vi "cDAQ_VI_Leo_Modified.vi"() -> ()   [LabVIEW 2022 SP3]
uses:
  <vilib>/Analysis/3filter.llb/Filter Passband Type.ctl
  <vilib>/Analysis/baseanly.llb/Mean (DBL).vi
  <vilib>/DAQmx/read.llb/DAQmx Read (Analog 1D Wfm NChan NSamp).vi
  STOP_GLOBAL.vi
  <vilib>/addons/control/pid/pid.llb/PID Lead-Lag (DBL).vi
  <vilib>/addons/control/pid/pid.llb/PID (DBL).vi
  <vilib>/DAQmx/configure/timing.llb/DAQmx Timing (Sample Clock).vi
  <vilib>/DAQmx/miscellaneous.llb/DAQmx Fill In Error Info.vi
  <vilib>/Analysis/3filter.llb/Butterworth Filter (DBL).vi
  <vilib>/Analysis/NI_AALBase.lvlib
  <vilib>/addons/control/pid/NI_PID_pid.lvlib
panel:
  out "Supply Pressure Mean":dbl format="%0.2f"
  out "Servo Voltage Input 3":cluster{dbl[], "Filtered X":dbl[]}[](graph)
  out "Servo Voltage Input 2":cluster{dbl[], dbl[]}(graph)
  out "Test":dynamicdata(graph)
  out "output":dbl format="%.2f"
  out "Voltage Input":dynamicdata(graph)
  out "Servo Voltage Input":cluster{dbl[], dbl[]}(graph)
  out "Elapsed Time (s)":dbl
  in  "Tab Control":T1(tab)
  in  "Channel Array":dbl[](array[numeric]) format="%_3g"
  out "error out 5":errorcluster
  in  "stop":bool
  out "Output":dbl(slide) scale=0.0..5.067
  out "elapsed time (s)":dbl format="%.3f"
  in  "reinitialize? (F)":bool
  out "Waveform Chart 2":cluster{"setpoint":dbl, dbl}(graph) caption="Waveform Chart"
  out "XY Graph":cluster{dbl[], dbl[]}[](graph)
  out "error out":errorcluster
  out "Steps on Needle 3":dbl[](array[numeric])
  in  "Error":dbl
  in  "Scaling Factor":dbl
  in  "x0":dbl
  in  "PID gains":T2={"proportional gain (Kc)"=1.0, "integral time (Ti, min)"=0.01, "derivative time (Td, min)"=0.0} {"derivative time (Td, min)" format="%.3f"; "integral time (Ti, min)" format="%.3f"; "proportional gain (Kc)" format="%.3f"}
  out "element":dbl
  out "Process variable":dbl
  out "Setpoint":dbl
  in  "setpoint profile":cluster{"time (s)":dbl, "setpoint":dbl}[](array[cluster]) {"setpoint" format="%.2f"; "time (s)" format="%.3f"}
  out "Steps on Servo":dbl[](array[numeric])
  out "Elapsed Time (s) 2":dbl caption="Elapsed Time (s)"
  out "HAS 3 SECONDS PASSED?":bool
  in  "PRESS TO START":bool
  out "All Channel Graph":cluster{dbl[], dbl[]}[](graph)
  out "Thrust":cluster{dbl[], dbl[]}(graph)
  out "Chamber Pressure":cluster{dbl[], dbl[]}(graph)
  out "Supply Pressure":cluster{dbl[], dbl[]}(graph)
  out "MassFlow":cluster{dbl[], dbl[]}(graph)
  out "Temperature":cluster{dbl[], dbl[]}(graph)
  out "error out 3":errorcluster caption="error out"
  out "error out 2":errorcluster
  in  "rate":dbl=1000.0 format="%0.2f"
  in  "number of samples":i32=100
  in  "File Format":string
  in  "File Name Out":string
  in  "Data Collection Folder":path
  out "Temperature":dynamicdata(graph)
  out "Numeric 2":i32
  out "Thrust lb":dynamicdata(graph)
  in  "Types of Testing":enum32{"Test Firing", "Cold Flow Rig"}(tab)
  out "Saving Data":bool
  out "Filename Out":path
  in  "Collect Data?":bool=TRUE caption="Enable"
  in  "Collect Data? 2":bool=TRUE caption="Enable"
  out "Saving Data":bool
  out "Filename Out":path
  out "Supply Pressure PSI":dynamicdata(graph)
  out "Mass Flow L/min":dynamicdata(graph)
  out "Chamber Pressure":dynamicdata(graph)
  # "Control Loop"
  # "DATA LOGGING INFORMATION"
  # "ANALOG VOLTAGE OUTPUT"
  # "RESULTS"
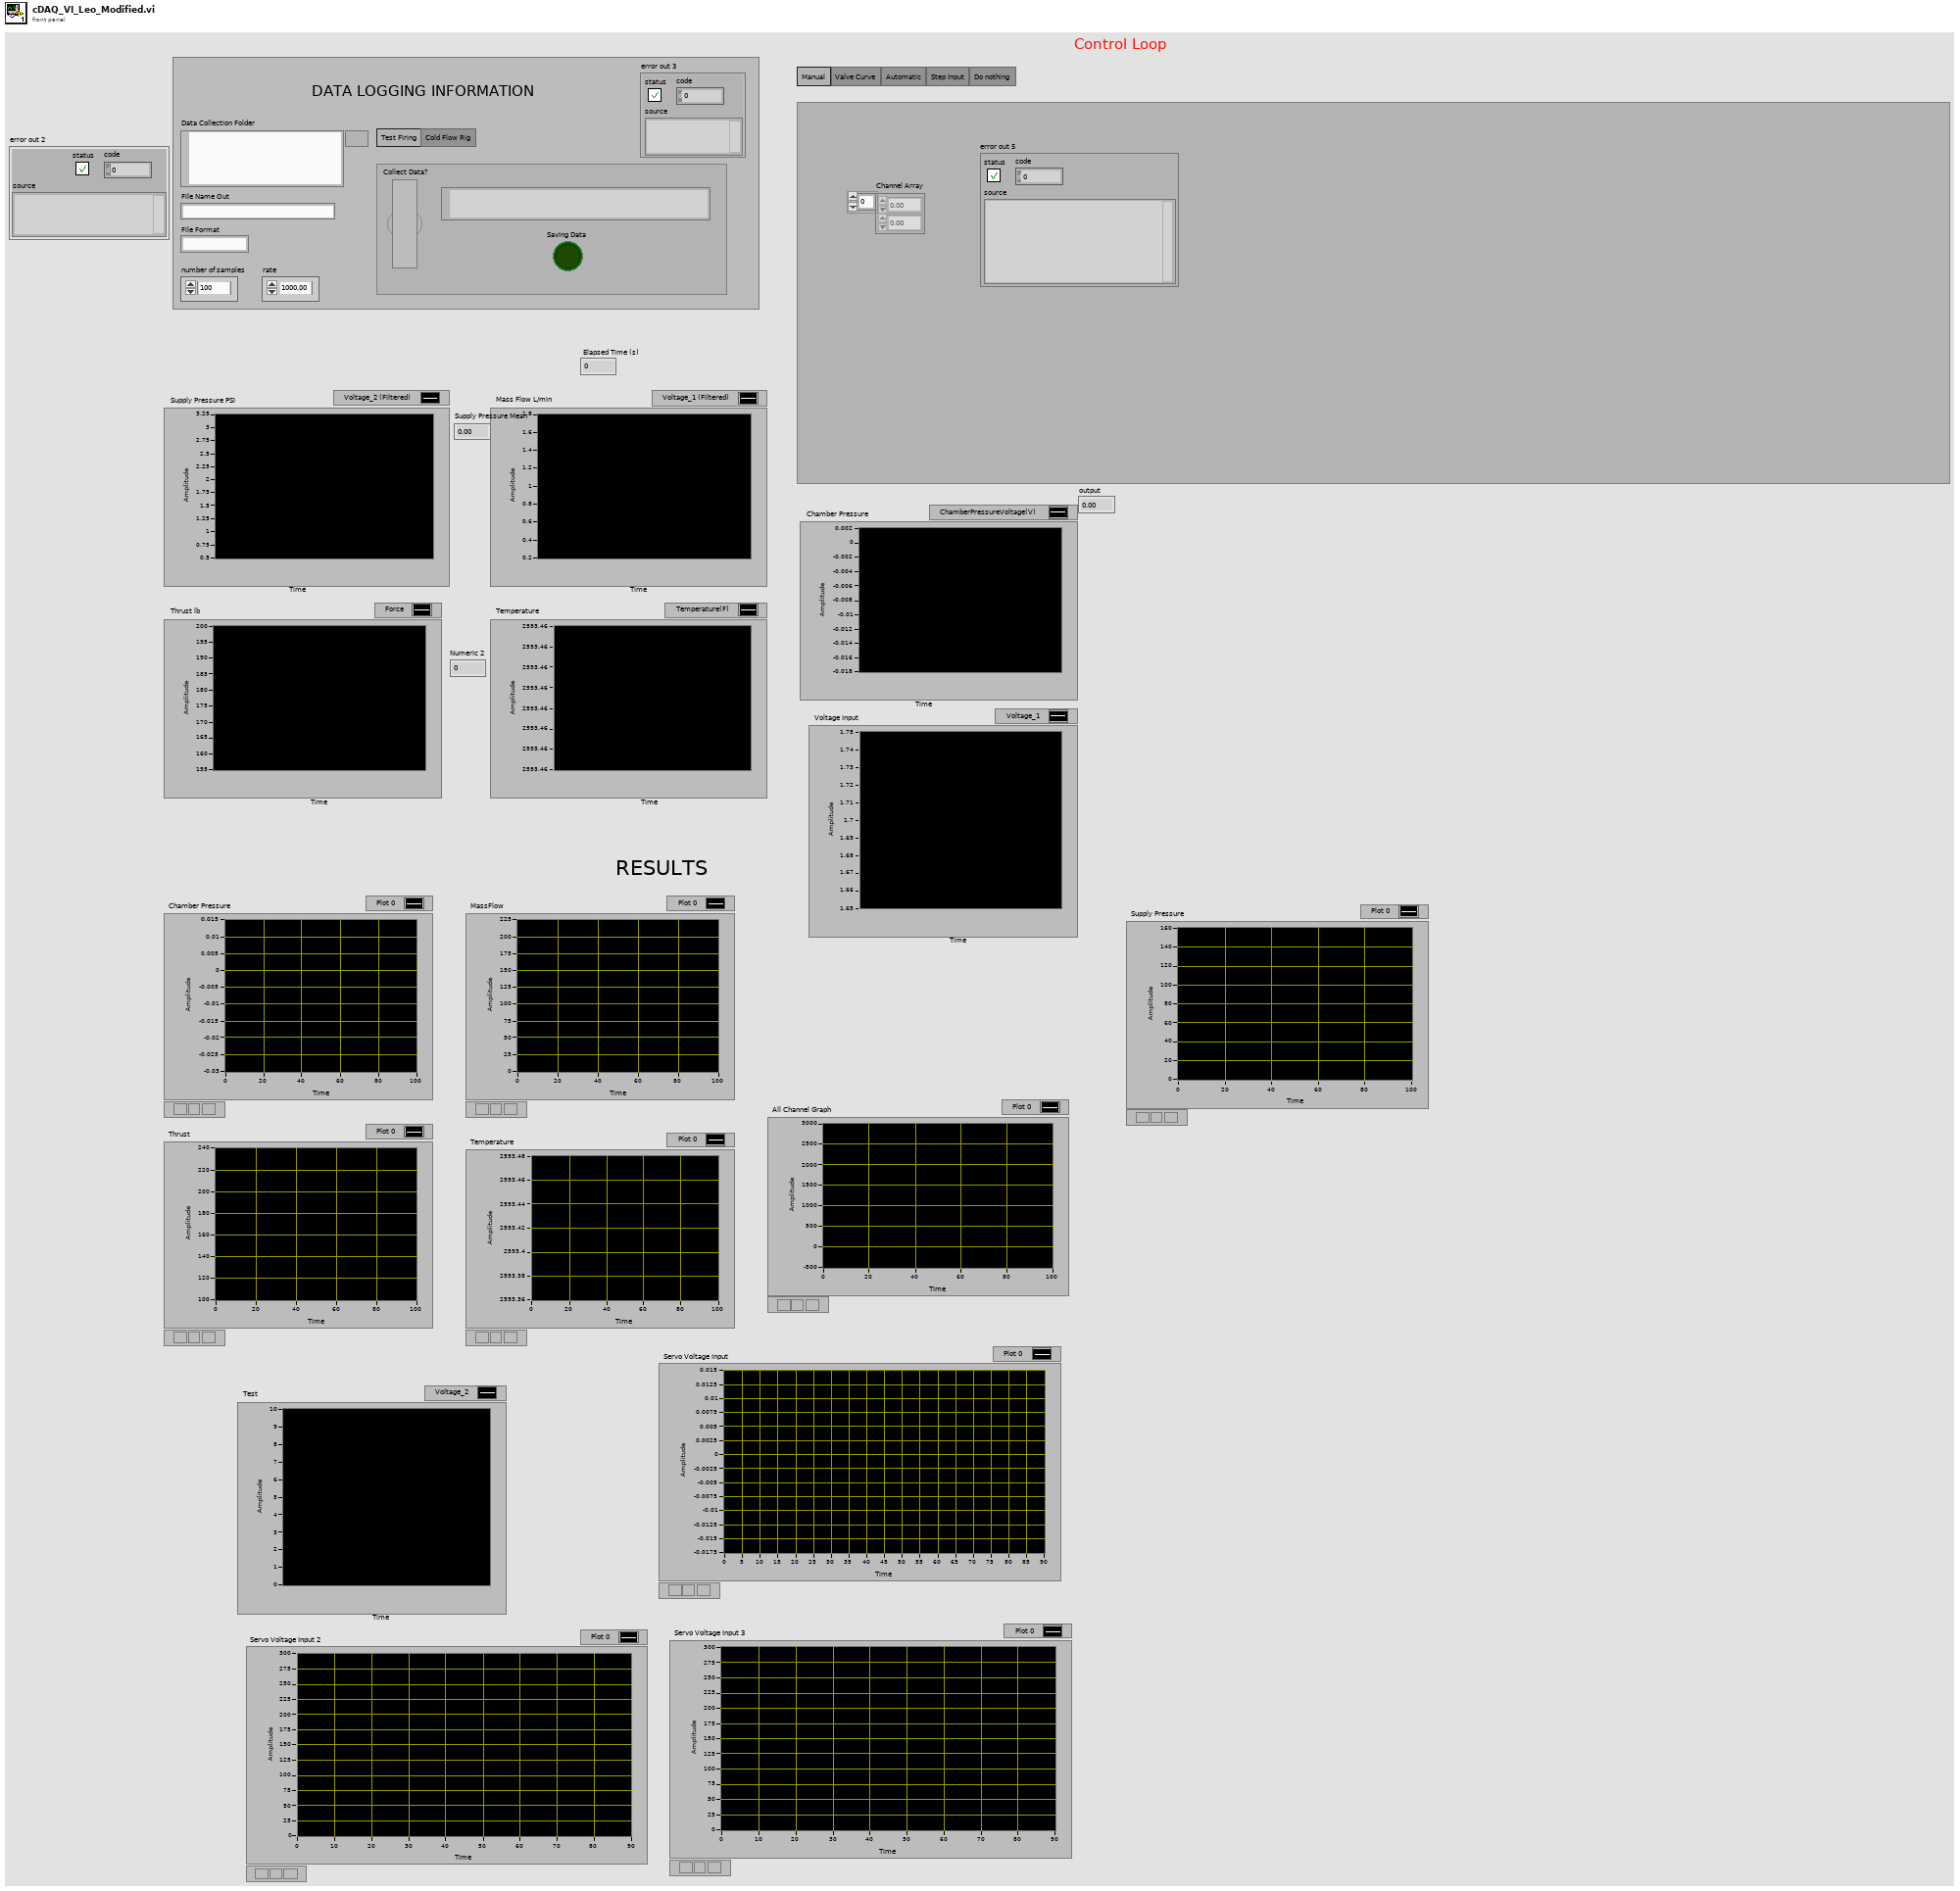
[diagram p1: front panel]
types:
  T1 = enum32{"Manual", "Valve Curve", "Automatic", "Step Input", "Do nothing"}
  T2 = cluster{"proportional gain (Kc)":dbl, "integral time (Ti, min)":dbl, "derivative time (Td, min)":dbl}
  T3 = typedef "NI_AALBase.lvlib/Filter Passband Type.ctl" = enum32{"Lowpass", "Highpass", "Bandpass", "Bandstop"}
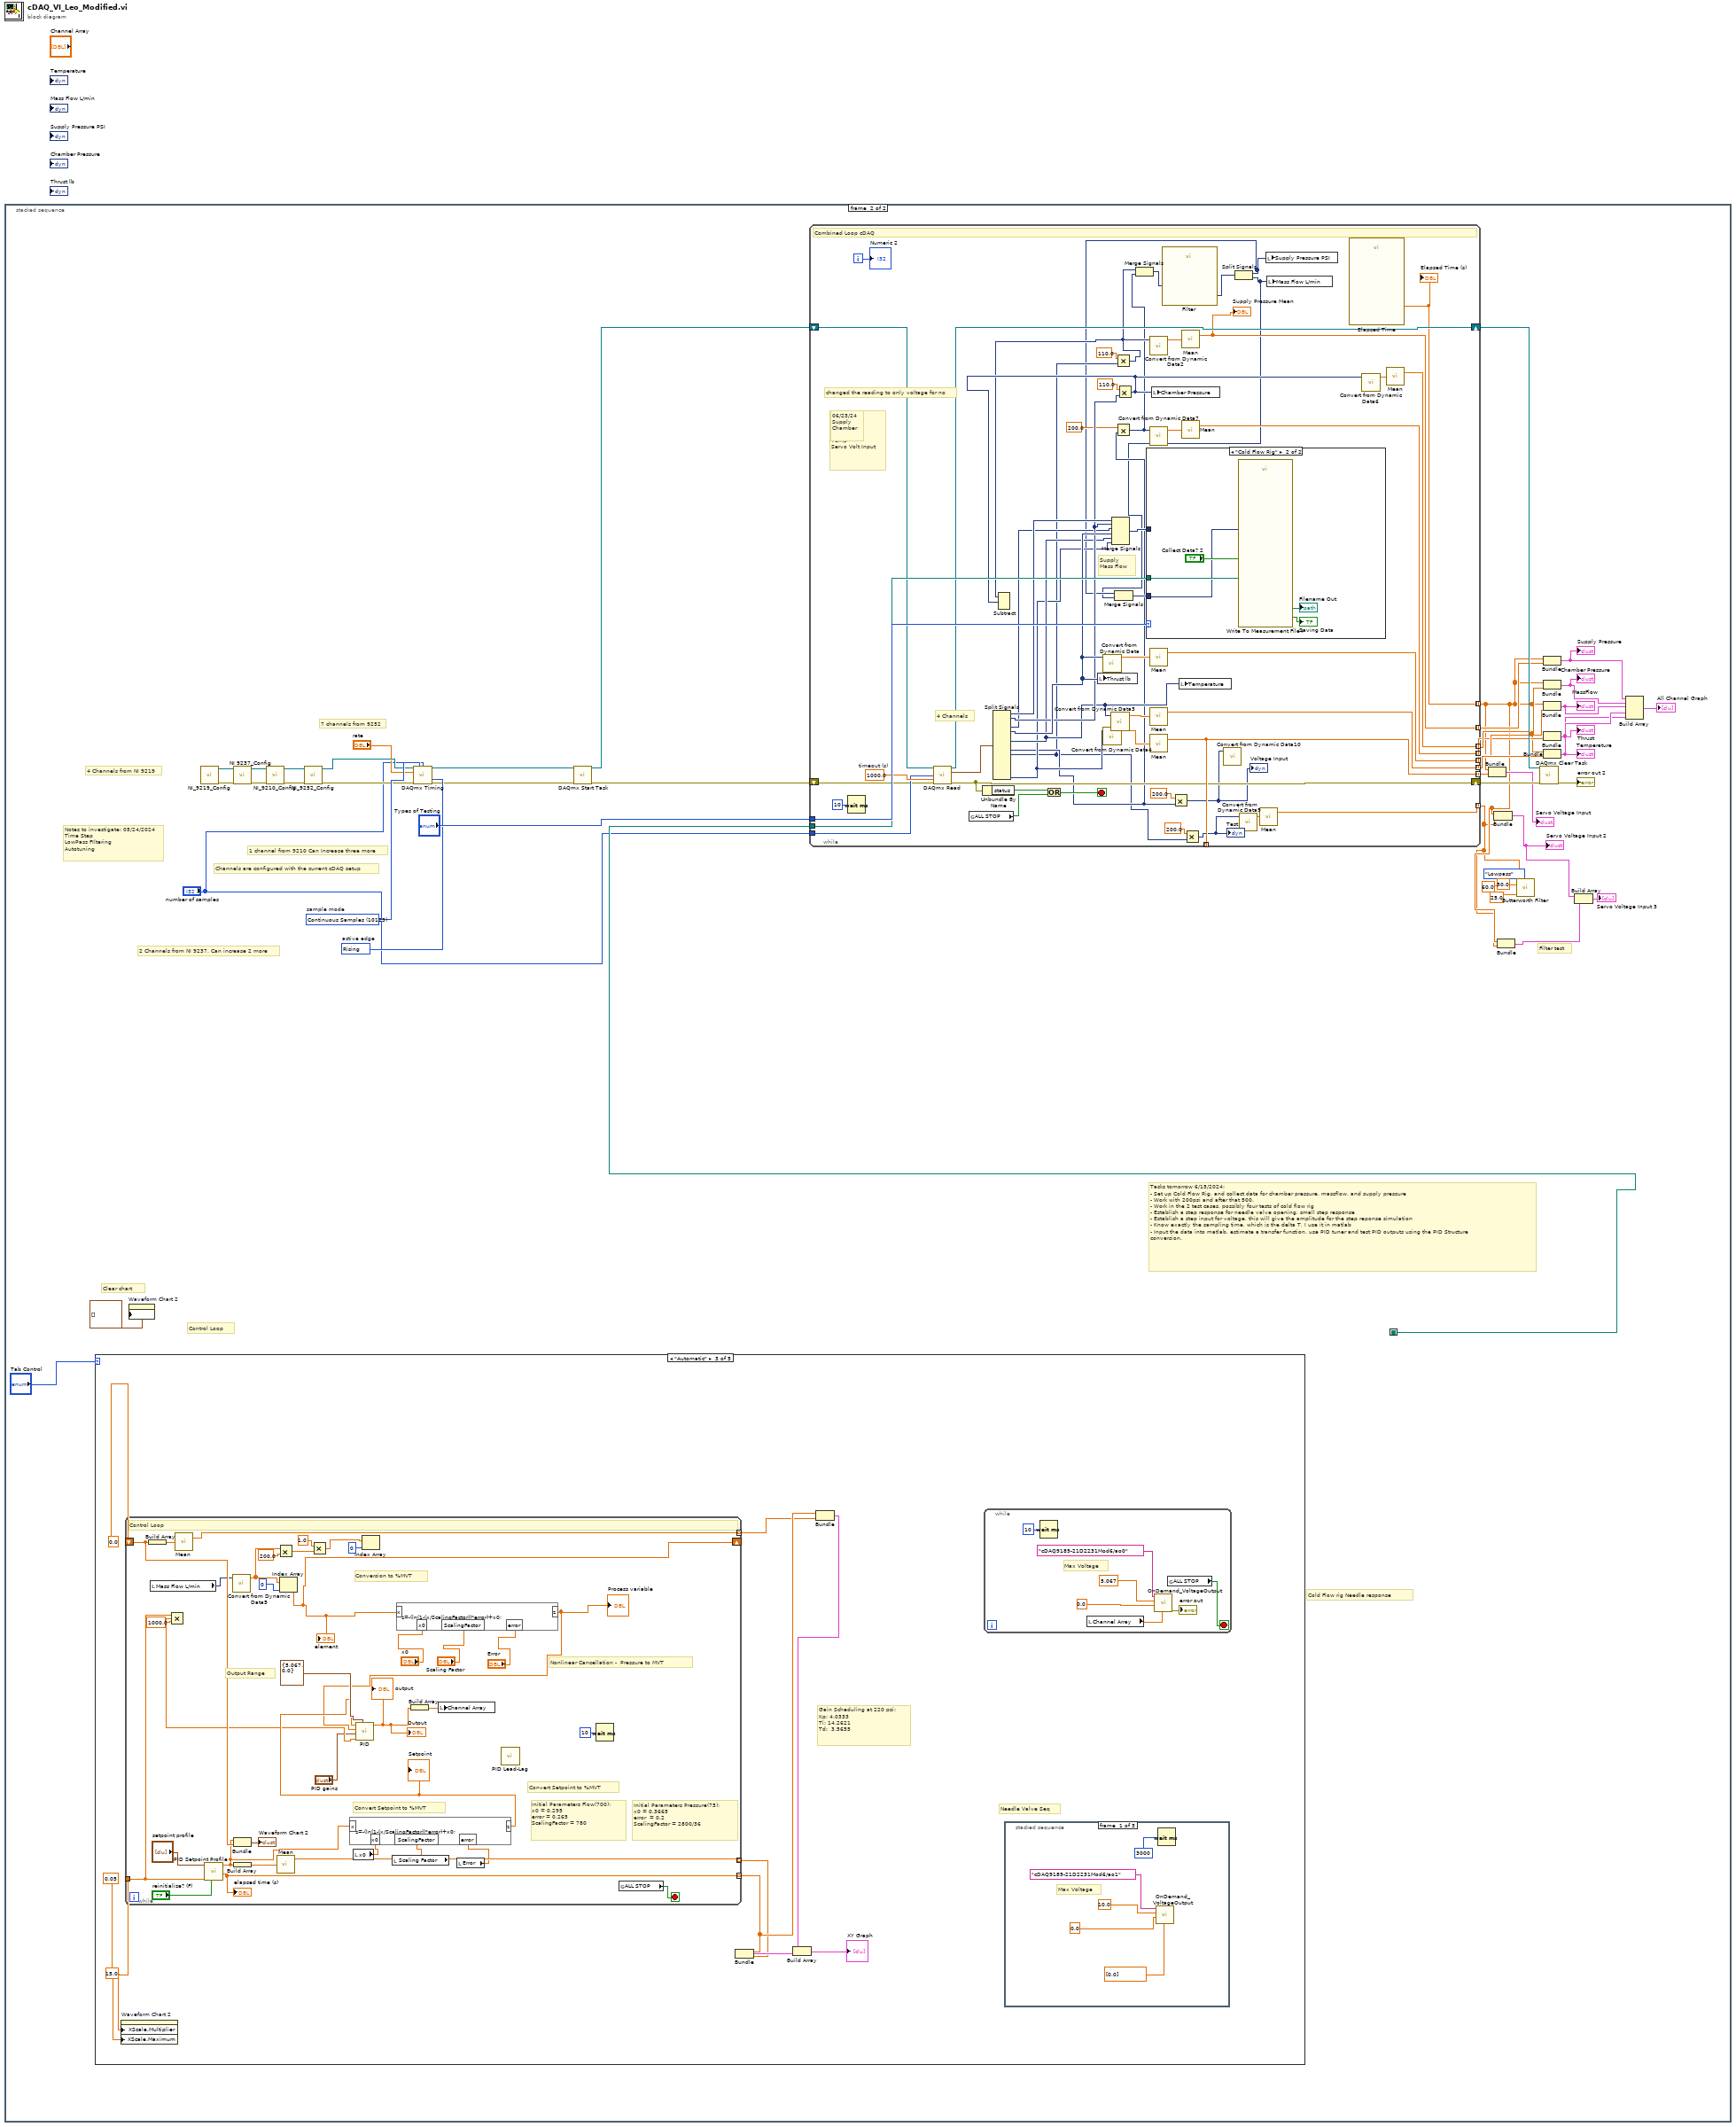
[diagram p0: block diagram]
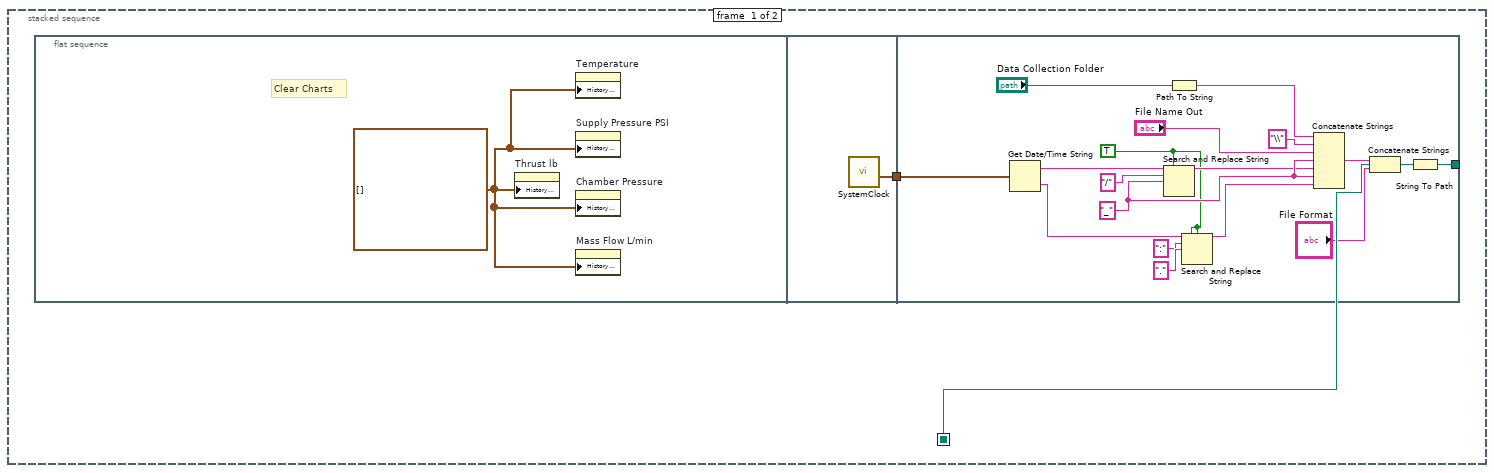
[diagram p2: hidden frame]
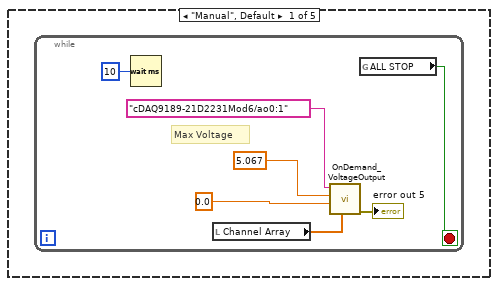
[diagram p3: hidden frame]
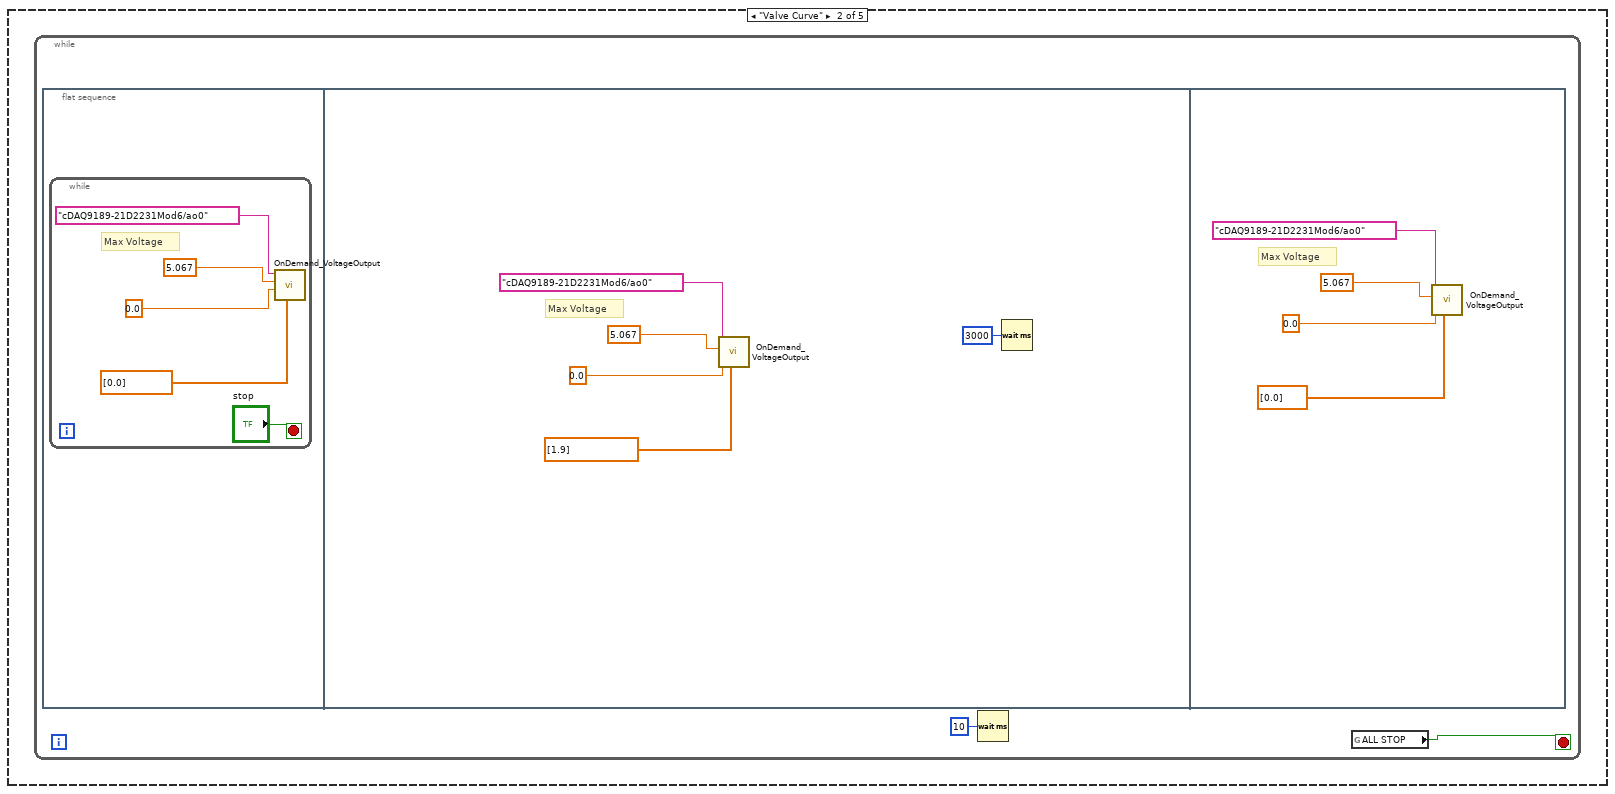
[diagram p4: hidden frame]
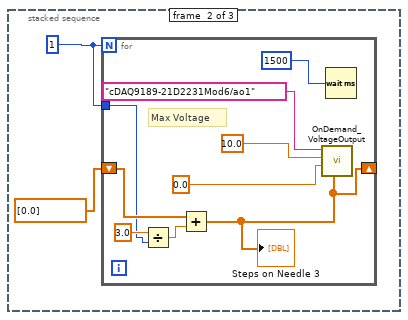
[diagram p5: hidden frame]
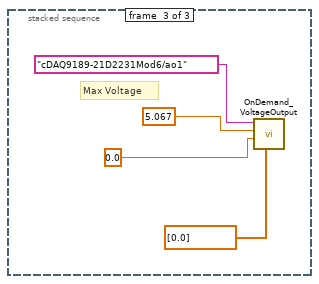
[diagram p6: hidden frame]
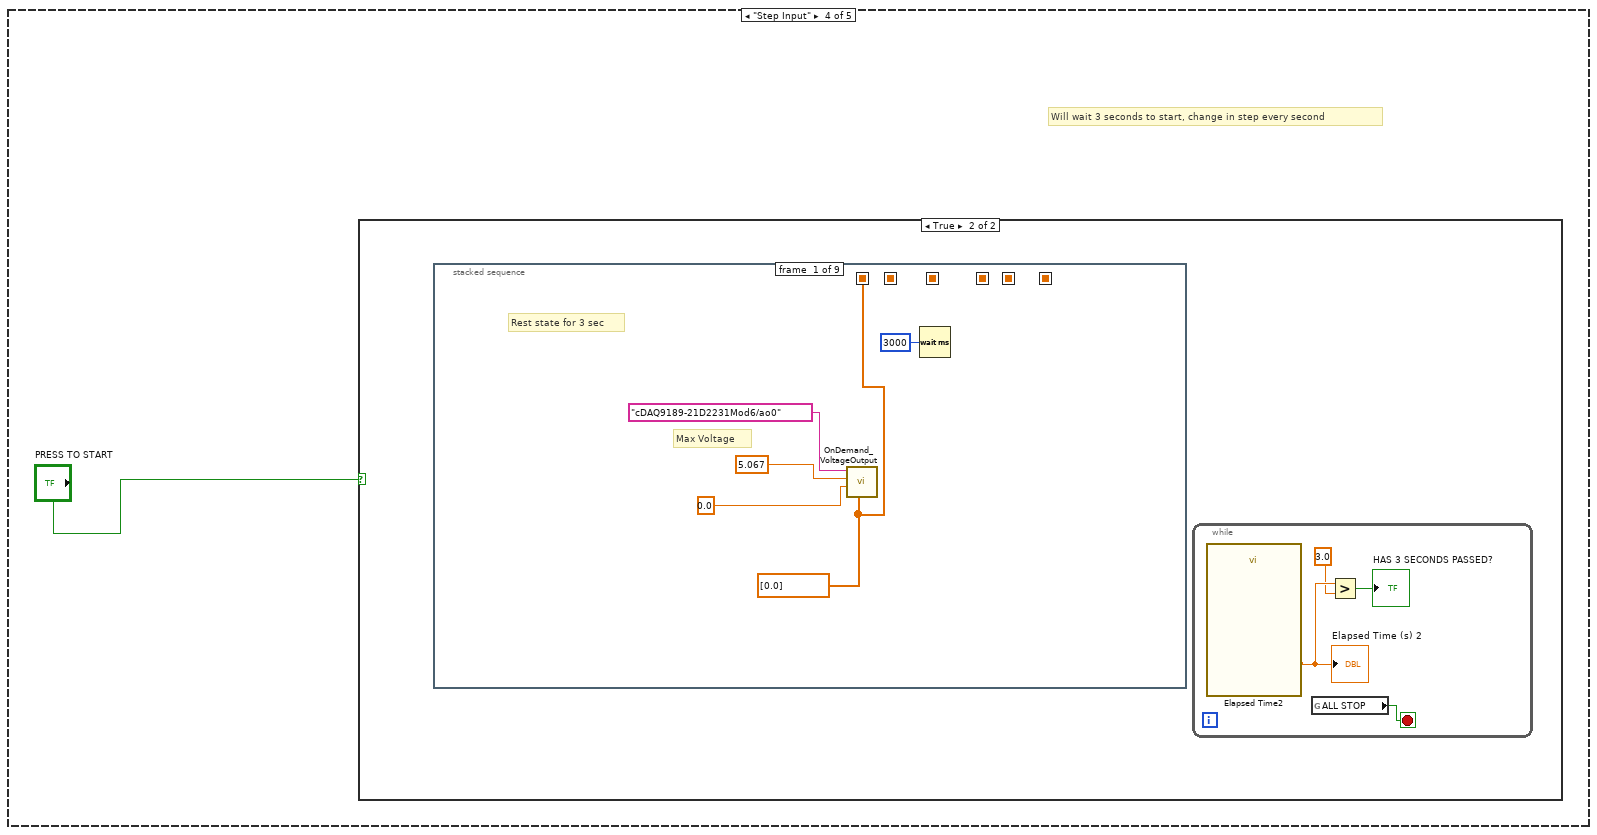
[diagram p7: hidden frame]
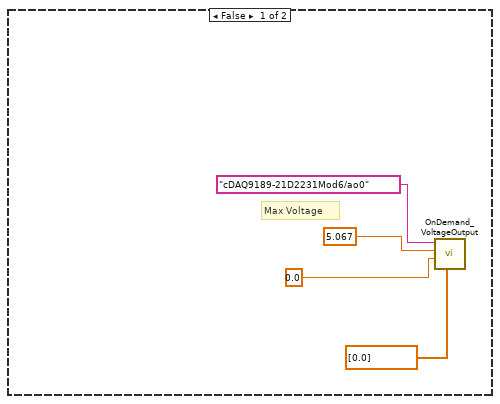
[diagram p8: hidden frame]
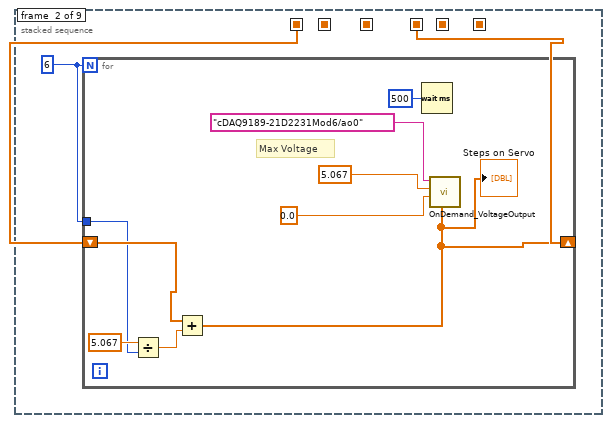
[diagram p9: hidden frame]
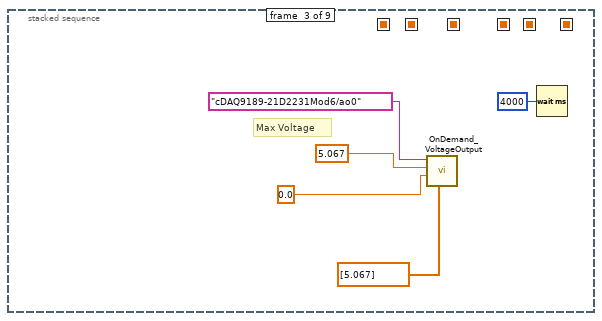
[diagram p10: hidden frame]
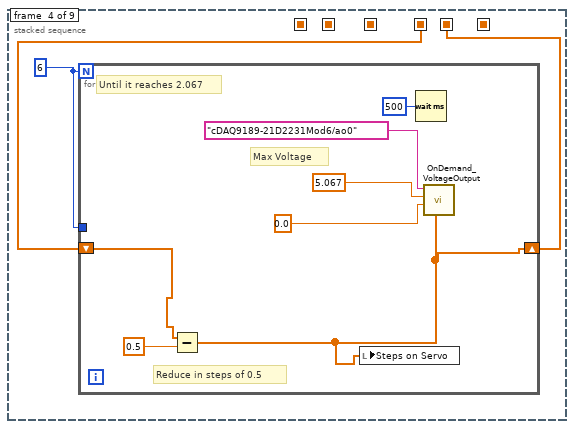
[diagram p11: hidden frame]
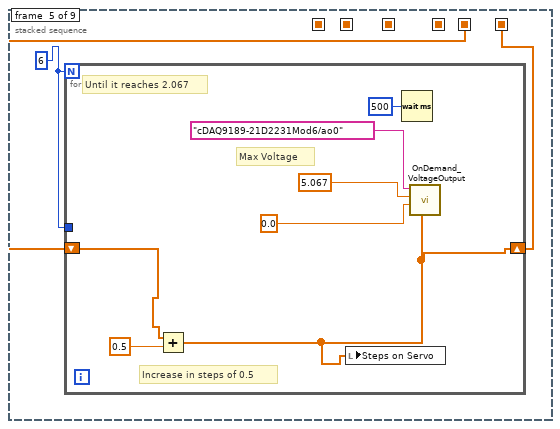
[diagram p12: hidden frame]
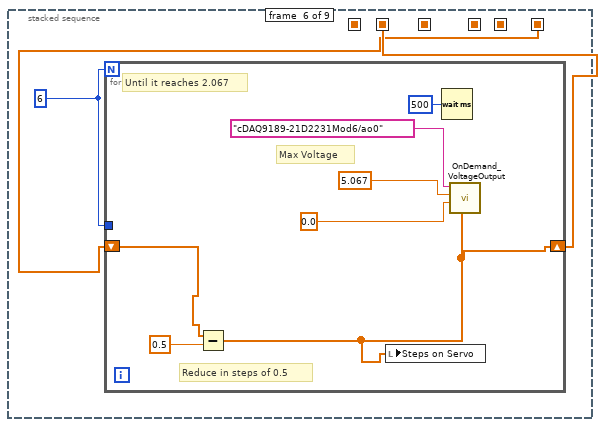
[diagram p13: hidden frame]
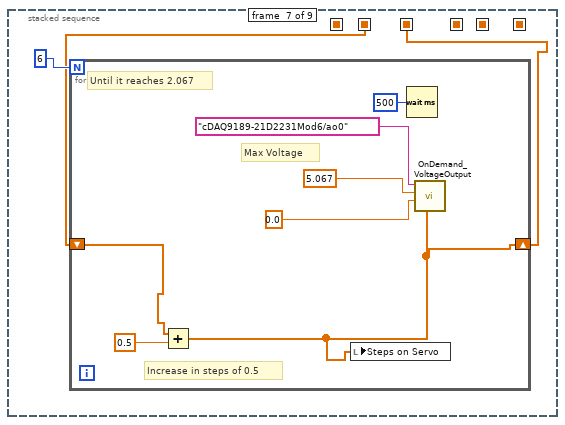
[diagram p14: hidden frame]
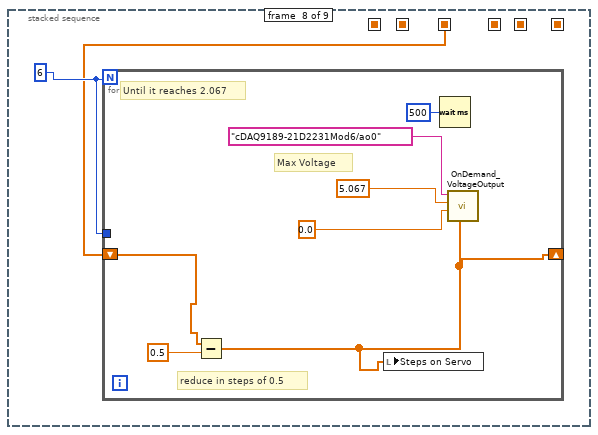
[diagram p15: hidden frame]
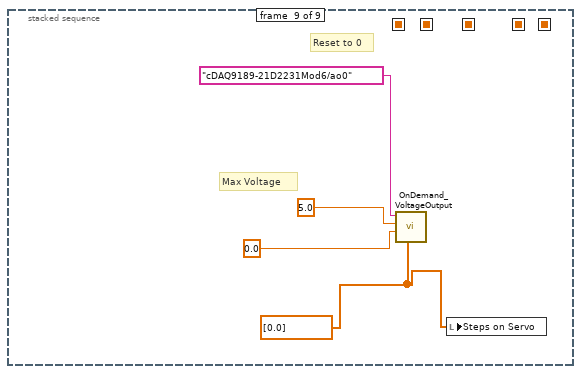
[diagram p16: hidden frame]
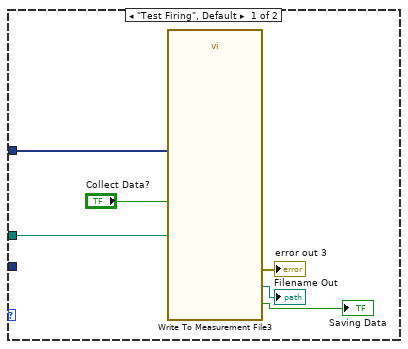
[diagram p18: hidden frame]
diagram:
  n1 = stacked-sequence {
    seq-local: [w1 _] -> [_ w66]
    frame #0 {
      n2 = flat-sequence {
        tunnel: [w4] -> w2
        tunnel: w2 -> [w11]
        tunnel: [w10] -> w1
        frame #0 {
          w3 = waveform(dbl)[] []
          # "Clear Charts"
          n3 = property on="Thrust lb" class="WFChart (strict)"("History Data"=w3) -> ()  [unwired: 2 in, 2 out]
          n4 = property on="Temperature" class="WFChart (strict)"("History Data"=w3) -> ()  [unwired: 2 in, 2 out]
          n5 = property on="Supply Pressure PSI" class="WFChart (strict)"("History Data"=w3) -> ()  [unwired: 2 in, 2 out]
          n6 = property on="Chamber Pressure" class="WFChart (strict)"("History Data"=w3) -> ()  [unwired: 2 in, 2 out]
          n7 = property on="Mass Flow L/min" class="WFChart (strict)"("History Data"=w3) -> ()  [unwired: 2 in, 2 out]
        }
        frame #1 {
          n8 = call "SystemClock.vi"() -> ("LabVIEW Time Stamp"=w4:timestamp)  [unwired: 9 in, 2 out]
        }
        frame #2 {
          w6 = TRUE ("replace all? (F)")
          w19 = "_" ("string")
          n9 = Get Date/Time String(seconds (now)=w11) -> (date string=w13:string, time string=w16:string)  [unwired: 2 in]
          n10 = Search and Replace String(replace all?=w6, input string=w13, search string="/", replace string=w19) -> (result string=w15:string)  [unwired: 4 in, 3 out]
          n11 = Path To String(path="Data Collection Folder") -> (string=w8:string)
          n12 = Search and Replace String(replace all?=w6, case sensitive?=w6, input string=w16, search string=":", replace string="." ("replace string (\"\")")) -> (result string=w20:string)  [unwired: 3 in, 3 out]
          n13 = Concatenate Strings(w8, "\\" ("string"), "File Name Out", w19, w15, w19, w20) -> (w21:string)
          n14 = Concatenate Strings(w21, "File Format") -> (w22:string)
          n15 = String To Path(string=w22) -> (path=w10:path)
        }
      }
    }
    frame #1 {
      w64 = 10123 items=["Finite Samples"=10178, "Continuous Samples"=10123, "Hardware Timed Single Point"=12522]  # sample mode
      w65 = 10280 items=["Rising"=10280, "Falling"=10171]  # active edge
      # "Filter test"
      # "Cold Flow rig Needle response"
      # "Tasks tomorrow 6/15/2024:\n- Set up Cold Flow Rig, and collect data for chamber pressure, massflow, and supply pressure\n- Work with 200psi and after that 500.\n- Work in the 2 test cases, possibly four tests of cold flow rig\n- Establish a step response for needle valve opening, small step response\n- Establish a step input for voltage, this will give the amplitude for the step reponse simulation\n- Know exactly the sampling time, which is the delta T, I use it in matlab\n- Input the data into matlab, estimate a transfer function, use PID tuner and test PID outputs using the PID Structure\nconversion."
      # "Control Loop"
      # "Clear chart"
      # "Notes to investigate: 05/24/2024\nTime Step\nLowPass FIltering\nAutotuning"
      # "Channels are configured with the current cDAQ setup"
      # "7 channels from 9252"
      # "1 channel from 9210 Can Increase three more"
      # "2 Channels from NI 9237, Can increase 2 more"
      # "4 Channels from NI 9219"
      n16 = case shown="\"Automatic\"" "Tab Control" {
        frame "Manual", Default {
          n17 = while {
            stop <- w74 stop-if-true
            # "Max Voltage"
            n18 = Wait (ms)(milliseconds to wait=u32 10) -> ()  [unwired: 1 out]
            n19 = local read "Channel Array"() -> (w70:dbl[])
            n20 = call "OnDemand_VoltageOutput.vi"("Channel Array"=w70, "minimum voltage"=0.0, "maximum voltage"=5.067, "physical channels"="cDAQ9189-21D2231Mod6/ao0:1") -> ("error out"=→"error out 5":errorcluster)  [unwired: 7 in]
            n21 = global read "STOP_GLOBAL.vi" "ALL STOP"() -> (w74:bool)
          }
        }
        frame "Valve Curve" {
          n22 = while {
            stop <- w75 stop-if-true
            n23 = flat-sequence {
              frame #0 {
                n24 = while {
                  stop <- "stop" stop-if-true
                  # "Max Voltage"
                  n25 = call "OnDemand_VoltageOutput.vi"("Channel Array"=dbl[] [0.0], "minimum voltage"=0.0, "maximum voltage"=5.067, "physical channels"="cDAQ9189-21D2231Mod6/ao0") -> ()  [unwired: 7 in, 1 out]
                }
              }
              frame #1 {
                # "Max Voltage"
                n26 = call "OnDemand_VoltageOutput.vi"("Channel Array"=dbl[] [1.9], "minimum voltage"=0.0, "maximum voltage"=5.067, "physical channels"="cDAQ9189-21D2231Mod6/ao0") -> ()  [unwired: 7 in, 1 out]
                n27 = Wait (ms)(milliseconds to wait=u32 3000) -> ()  [unwired: 1 out]
              }
              frame #2 {
                # "Max Voltage"
                n28 = call "OnDemand_VoltageOutput.vi"("Channel Array"=dbl[] [0.0], "minimum voltage"=0.0, "maximum voltage"=5.067, "physical channels"="cDAQ9189-21D2231Mod6/ao0") -> ()  [unwired: 7 in, 1 out]
              }
            }
            n29 = Wait (ms)(milliseconds to wait=u32 10) -> ()  [unwired: 1 out]
            n30 = global read "STOP_GLOBAL.vi" "ALL STOP"() -> (w75:bool)
          }
        }
        frame "Automatic" {
          w99 = 0.05 ("dt (s)")
          # "Gain Scheduling at 220 psi:\nKp: 4.0333\nTi: 14.2621\nTd:  3.5655"
          # "Needle Valve Seq"
          n31 = property on="Waveform Chart 2" class="WFChart (strict)"("XScale.Multiplier"=w99, "XScale.Maximum"=15.0 ("X Scale.Range:Maximum")) -> ()  [unwired: 2 in, 2 out]
          n32 = while {
            shift-right: [w134] -> _
            shift-left: 0.0 -> [w152]
            tunnel: w99 -> [w155]
            tunnel: [w153] -> w94 mode=indexing
            tunnel: [w151] -> w92 mode=indexing
            tunnel: [w149] -> w93 mode=indexing
            stop <- w162 stop-if-true
            # "Initial Parameters Pressure(75):\nx0 = 0.3665\nerror  = 0.2\nScalingFactor = 2800/36"
            # "Initial Parameters Flow(700):\nx0 = 0.295\nerror = 0.265\nScalingFactor = 780"
            # "Convert Setpoint to %MVT"
            # "Nonlinear Cancellation -  Pressure to MVT"
            # "Convert Setpoint to %MVT"
            # "Conversion to %MVT"
            # "Output Range"
            # "Control Loop"
            n33 = Build Array(w152) -> (w150:dbl[])
            n34 = local read "Mass Flow L/min"() -> (w131:dynamicdata)
            n35 = Multiply(x=w155, y=1000.0) -> (x*y=w138:dbl)
            n36 = call-poly <vilib>:"Mean.vi"("X"=w150) -> ("mean"=w151:dbl)  [unwired: 1 out]
            n37 = call <vilib>:"PID Setpoint Profile.vi"("reinitialize? (F)"="reinitialize? (F)", "dt (s)"=w155, "setpoint profile"="setpoint profile") -> ("elapsed time (s)"=w153:dbl, "setpoint"=w145:dbl)  [unwired: 3 in, 2 out]
            "elapsed time (s)" <- w153
            n38 = call "Convert from Dynamic Data5"("Dynamic Data Type"=w131) -> ("Array"=w132:dbl[])  [unwired: 3 in]
            n39 = Bundle("setpoint"=w145, w152) -> (→"Waveform Chart 2":cluster{"setpoint":dbl, dbl})  [unwired: 1 in]
            n40 = Build Array(w145) -> (w146:dbl[])
            n41 = Multiply(x=w132, y=200.0 ("x")) -> (x*y=w133:dbl[])
            n42 = call-poly <vilib>:"Mean.vi"("X"=w146) -> ("mean"=w149:dbl)  [unwired: 1 out]
            n43 = Index Array(array=w132, index=0) -> (element=w134:dbl)
            "element" <- w134
            n44 = Multiply(x=1.0, y=w133) -> (x*y=w160:dbl[])
            n45 = local read "x0"() -> (w144:dbl)
            n46 = Index Array(array=w160, index=0) -> ()  [unwired: 1 out]
            n47 = local read "Scaling Factor"() -> (w143:dbl)
            n48 = formula code="z=-(ln(1-(x/ScalingFactor))*error)+x0;"("x"=w134, "x0"="x0", "ScalingFactor"="Scaling Factor", "error"="Error") -> ("z"=w129:dbl)
            "Process variable" <- w129
            n49 = local read "Error"() -> (w142:dbl)
            n50 = formula code="z=-(ln(1-(x/ScalingFactor))*error)+x0;"("x"=w145, "x0"=w144, "ScalingFactor"=w143, "error"=w142) -> ("z"=w139:dbl)
            "Setpoint" <- w139
            n51 = call-poly <vilib>:"PID.vi"("output range"=cluster{"output high":dbl, "output low":dbl} {"output high"=5.067, "output low"=0.0}, "dt (s)"=w138, "PID gains"="PID gains", "process variable"=w129, "setpoint"=w139) -> ("output"=w141:dbl)  [unwired: 5 in, 1 out]
            "Output" <- w141
            "output" <- w141
            n52 = Build Array(w141) -> (w154:dbl[])
            n53 = local write "Channel Array"(w154) -> ()
            n54 = call-poly <vilib>:"PID Lead-Lag.vi"() -> ()  [unwired: 8 in, 2 out]
            n55 = Wait (ms)(milliseconds to wait=u32 10) -> ()  [unwired: 1 out]
            n56 = global read "STOP_GLOBAL.vi" "ALL STOP"() -> (w162:bool)
          }
          n57 = Bundle(w94, w93) -> (w96:cluster{dbl[], dbl[]})  [unwired: 1 in]
          n58 = Bundle(w94, w92) -> (w95:cluster{dbl[], dbl[]})  [unwired: 1 in]
          n59 = Build Array(w95, w96) -> (→"XY Graph":cluster{dbl[], dbl[]}[])
          n60 = while {
            stop <- w126 stop-if-true
            # "Max Voltage"
            n61 = Wait (ms)(milliseconds to wait=u32 10) -> ()  [unwired: 1 out]
            n62 = local read "Channel Array"() -> (w122:dbl[])
            n63 = call "OnDemand_VoltageOutput.vi"("Channel Array"=w122, "minimum voltage"=0.0, "maximum voltage"=5.067, "physical channels"="cDAQ9189-21D2231Mod6/ao0") -> ("error out"=→"error out":errorcluster)  [unwired: 7 in]
            n64 = global read "STOP_GLOBAL.vi" "ALL STOP"() -> (w126:bool)
          }
          n65 = stacked-sequence {
            frame #0 {
              # "Max Voltage"
              n66 = call "OnDemand_VoltageOutput.vi"("Channel Array"=dbl[] [0.0], "minimum voltage"=0.0, "maximum voltage"=10.0, "physical channels"="cDAQ9189-21D2231Mod6/ao1") -> ()  [unwired: 7 in, 1 out]
              n67 = Wait (ms)(milliseconds to wait=u32 3000) -> ()  [unwired: 1 out]
            }
            frame #1 {
              w105 = 1
              n68 = for {
                N: w105 -> [_]
                shift-right: [w107] -> _
                shift-left: dbl[] [0.0] -> [w111]
                tunnel: w105 -> [w109]
                # "Max Voltage"
                n69 = Divide(x=3.0, y=w109) -> (x/y=w108:dbl)
                n70 = Add(x=w111, y=w108) -> (x+y=w107:dbl[])
                "Steps on Needle 3" <- w107
                n71 = call "OnDemand_VoltageOutput.vi"("Channel Array"=w107, "minimum voltage"=0.0, "maximum voltage"=10.0, "physical channels"="cDAQ9189-21D2231Mod6/ao1") -> ()  [unwired: 7 in, 1 out]
                n72 = Wait (ms)(milliseconds to wait=u32 1500) -> ()  [unwired: 1 out]
              }
            }
            frame #2 {
              # "Max Voltage"
              n73 = call "OnDemand_VoltageOutput.vi"("Channel Array"=dbl[] [0.0], "minimum voltage"=0.0, "maximum voltage"=5.067, "physical channels"="cDAQ9189-21D2231Mod6/ao1") -> ()  [unwired: 7 in, 1 out]
            }
          }
        }
        frame "Step Input" {
          # "Will wait 3 seconds to start, change in step every second"
          n74 = case shown="True" "PRESS TO START" {
            frame False {
              # "Max Voltage"
              n75 = call "OnDemand_VoltageOutput.vi"("Channel Array"=dbl[] [0.0], "minimum voltage"=0.0, "maximum voltage"=5.067, "physical channels"="cDAQ9189-21D2231Mod6/ao0") -> ()  [unwired: 7 in, 1 out]
            }
            frame True {
              n76 = stacked-sequence {
                seq-local: [_ _ _ _ _ w215 _ _ _] -> [_ _ _ _ _ _ w225 _ _]
                seq-local: [_ _ _ _ _ _ w224 _ _] -> [_ _ _ _ _ _ _ w234 _]
                seq-local: [w172 _ _ _ _ _ _ _ _] -> [_ w178 _ _ _ _ _ _ _]
                seq-local: [_ w177 _ _ _ _ _ _ _] -> [_ _ _ w195 _ _ _ _ _]
                seq-local: [_ _ _ w194 _ _ _ _ _] -> [_ _ _ _ w205 _ _ _ _]
                seq-local: [_ _ _ _ w204 _ _ _ _] -> [_ _ _ _ _ w214 _ _ _]
                frame #0 {
                  w172 = dbl[] [0.0]
                  # "Rest state for 3 sec"
                  # "Max Voltage"
                  n77 = call "OnDemand_VoltageOutput.vi"("Channel Array"=w172, "minimum voltage"=0.0, "maximum voltage"=5.067, "physical channels"="cDAQ9189-21D2231Mod6/ao0") -> ()  [unwired: 7 in, 1 out]
                  n78 = Wait (ms)(milliseconds to wait=u32 3000) -> ()  [unwired: 1 out]
                }
                frame #1 {
                  w179 = 6
                  n79 = for {
                    N: w179 -> [_]
                    shift-right: [w180] -> w177
                    shift-left: w178 -> [w187]
                    tunnel: w179 -> [w181]
                    # "Max Voltage"
                    n80 = Divide(x=5.067, y=w181) -> (x/y=w183:dbl)
                    n81 = Add(x=w187, y=w183) -> (x+y=w180:dbl[])
                    "Steps on Servo" <- w180
                    n82 = Wait (ms)(milliseconds to wait=u32 500) -> ()  [unwired: 1 out]
                    n83 = call "OnDemand_VoltageOutput.vi"("Channel Array"=w180, "minimum voltage"=0.0, "maximum voltage"=5.067, "physical channels"="cDAQ9189-21D2231Mod6/ao0") -> ()  [unwired: 7 in, 1 out]
                  }
                }
                frame #2 {
                  # "Max Voltage"
                  n84 = call "OnDemand_VoltageOutput.vi"("Channel Array"=dbl[] [5.067], "minimum voltage"=0.0, "maximum voltage"=5.067, "physical channels"="cDAQ9189-21D2231Mod6/ao0") -> ()  [unwired: 7 in, 1 out]
                  n85 = Wait (ms)(milliseconds to wait=u32 4000) -> ()  [unwired: 1 out]
                }
                frame #3 {
                  w196 = 6
                  n86 = for {
                    N: w196 -> [_]
                    shift-right: [w197] -> w194
                    shift-left: w195 -> [w203]
                    tunnel: w196 -> [_]
                    # "Max Voltage"
                    # "Until it reaches 2.067"
                    # "Reduce in steps of 0.5"
                    n87 = Subtract(x=w203, y=0.5) -> (x-y=w197:dbl[])
                    n88 = local write "Steps on Servo"(w197) -> ()
                    n89 = Wait (ms)(milliseconds to wait=u32 500) -> ()  [unwired: 1 out]
                    n90 = call "OnDemand_VoltageOutput.vi"("Channel Array"=w197, "minimum voltage"=0.0, "maximum voltage"=5.067, "physical channels"="cDAQ9189-21D2231Mod6/ao0") -> ()  [unwired: 7 in, 1 out]
                  }
                }
                frame #4 {
                  w206 = 6
                  n91 = for {
                    N: w206 -> [_]
                    shift-right: [w207] -> w204
                    shift-left: w205 -> [w213]
                    tunnel: w206 -> [_]
                    # "Max Voltage"
                    # "Until it reaches 2.067"
                    # "Increase in steps of 0.5"
                    n92 = Add(x=w213, y=0.5) -> (x+y=w207:dbl[])
                    n93 = local write "Steps on Servo"(w207) -> ()
                    n94 = Wait (ms)(milliseconds to wait=u32 500) -> ()  [unwired: 1 out]
                    n95 = call "OnDemand_VoltageOutput.vi"("Channel Array"=w207, "minimum voltage"=0.0, "maximum voltage"=5.067, "physical channels"="cDAQ9189-21D2231Mod6/ao0") -> ()  [unwired: 7 in, 1 out]
                  }
                }
                frame #5 {
                  w216 = 6
                  n96 = for {
                    N: w216 -> [_]
                    shift-right: [w217] -> w215
                    shift-left: w214 -> [w223]
                    tunnel: w216 -> [_]
                    # "Max Voltage"
                    # "Until it reaches 2.067"
                    # "Reduce in steps of 0.5"
                    n97 = Subtract(x=w223, y=0.5) -> (x-y=w217:dbl[])
                    n98 = local write "Steps on Servo"(w217) -> ()
                    n99 = Wait (ms)(milliseconds to wait=u32 500) -> ()  [unwired: 1 out]
                    n100 = call "OnDemand_VoltageOutput.vi"("Channel Array"=w217, "minimum voltage"=0.0, "maximum voltage"=5.067, "physical channels"="cDAQ9189-21D2231Mod6/ao0") -> ()  [unwired: 7 in, 1 out]
                  }
                }
                frame #6 {
                  n101 = for {
                    N: 6 -> [_]
                    shift-right: [w227] -> w224
                    shift-left: w225 -> [w233]
                    # "Max Voltage"
                    # "Until it reaches 2.067"
                    # "Increase in steps of 0.5"
                    n102 = Add(x=w233, y=0.5) -> (x+y=w227:dbl[])
                    n103 = local write "Steps on Servo"(w227) -> ()
                    n104 = Wait (ms)(milliseconds to wait=u32 500) -> ()  [unwired: 1 out]
                    n105 = call "OnDemand_VoltageOutput.vi"("Channel Array"=w227, "minimum voltage"=0.0, "maximum voltage"=5.067, "physical channels"="cDAQ9189-21D2231Mod6/ao0") -> ()  [unwired: 7 in, 1 out]
                  }
                }
                frame #7 {
                  w235 = 6
                  n106 = for {
                    N: w235 -> [_]
                    shift-right: [w236] -> _
                    shift-left: w234 -> [w242]
                    tunnel: w235 -> [_]
                    # "Max Voltage"
                    # "Until it reaches 2.067"
                    # "reduce in steps of 0.5"
                    n107 = Subtract(x=w242, y=0.5) -> (x-y=w236:dbl[])
                    n108 = local write "Steps on Servo"(w236) -> ()
                    n109 = Wait (ms)(milliseconds to wait=u32 500) -> ()  [unwired: 1 out]
                    n110 = call "OnDemand_VoltageOutput.vi"("Channel Array"=w236, "minimum voltage"=0.0, "maximum voltage"=5.067, "physical channels"="cDAQ9189-21D2231Mod6/ao0") -> ()  [unwired: 7 in, 1 out]
                  }
                }
                frame #8 {
                  w243 = dbl[] [0.0]
                  # "Reset to 0"
                  # "Max Voltage"
                  n111 = call "OnDemand_VoltageOutput.vi"("Channel Array"=w243, "minimum voltage"=0.0, "maximum voltage"=5.0, "physical channels"="cDAQ9189-21D2231Mod6/ao0") -> ()  [unwired: 7 in, 1 out]
                  n112 = local write "Steps on Servo"(w243) -> ()
                }
              }
              n113 = while {
                stop <- w171 stop-if-true
                n114 = call "Elapsed Time2"() -> ("Elapsed Time (s)"=w169:dbl)  [unwired: 12 in, 7 out]
                "Elapsed Time (s) 2" <- w169
                n115 = global read "STOP_GLOBAL.vi" "ALL STOP"() -> (w171:bool)
                n116 = Greater?(x=w169, y=3.0 ("x")) -> (0:→"HAS 3 SECONDS PASSED?":bool)
              }
            }
          }
        }
        frame "Do nothing" {
        }
      }
      n117 = property on="Waveform Chart 2" class="WFChart (strict)"("History Data"=cluster{"setpoint":dbl, dbl}[] []) -> ()  [unwired: 2 in, 2 out]
      n118 = call "NI_9219_Config.vi"() -> ("error out"=w47:errorcluster, "task out"=w57:refnum<k21>)  [unwired: 10 in]
      n119 = call "NI 9237_Config.vi"("error in"=w47, "task in"=w57) -> ("error out"=w55:errorcluster, "task out"=w56:refnum<k21>)  [unwired: 8 in]
      n120 = call "NI_9210_Config.vi"("error in"=w55, "task in"=w56) -> ("error out"=w53:errorcluster, "task out"=w54:refnum<k21>)  [unwired: 8 in]
      n121 = call "NI_9252_Config.vi"("error in"=w53, "task in"=w54) -> ("error out"=w51:errorcluster, "task out"=w52:refnum<k21>)  [unwired: 8 in]
      n122 = call-poly <vilib>:"DAQmx Timing.vi"("task/channels in"=w52, "sample mode"=w64, "samples per channel"="number of samples", "rate"="rate", "active edge"=w65, "error in"=w51) -> ("task out"=w63:refnum<k21>, "error out"=w62:errorcluster)  [unwired: 8 in]
      n123 = call <vilib>:"DAQmx Start Task.vi"("task/channels in"=w63, "error in"=w62) -> ("task out"=w61:refnum<k21>, "error out"=w60:errorcluster)  [unwired: 12 in]
      n124 = while {
        tunnel: "Types of Testing" -> [w298]
        tunnel: [w296] -> w42 mode=indexing
        tunnel: w66 -> [w291]
        tunnel: "number of samples" -> [w289]
        shift-right: [w263] -> w58
        shift-left: w60 -> [w288]
        shift-right: [w286] -> w59
        shift-left: w61 -> [w287]
        tunnel: [w257] -> w44 mode=indexing
        tunnel: [w282] -> w43 mode=indexing
        tunnel: [w280] -> w45 mode=indexing
        tunnel: [w276] -> w46 mode=indexing
        tunnel: [w267] -> w48 mode=indexing
        tunnel: [w275] -> w27 mode=indexing
        tunnel: [w267] -> _ mode=indexing
        tunnel: [w264] -> w23 mode=indexing
        i -> [w299]
        stop <- w292 stop-if-true
        w294 = 1000.0  # timeout (s)
        # "4 Channels"
        # "Supply\nMass Flow"
        # "06/23/24\nSupply\nChamber"
        # "Supply\nChamber\nMassflow\nThrust\nTemp\nServo Volt Input"
        # "changed the reading to only voltage for no"
        # "Combined Loop cDAQ"
        n125 = Wait (ms)(milliseconds to wait=u32 10) -> ()  [unwired: 1 out]
        n126 = call-poly <vilib>:"DAQmx Read.vi"("task/channels in"=w287, "number of samples per channel"=w289, "timeout"=w294, "error in"=w288) -> ("task out"=w286:refnum<k21>, "data"=w290:waveform(dbl)[], "error out"=w263:errorcluster)  [unwired: 9 in]
        n127 = global read "STOP_GLOBAL.vi" "ALL STOP"() -> (w293:bool)
        n128 = Unbundle By Name(w263) -> ("status"=w295:bool)
        n129 = Split Signals(w290) -> (w272:dynamicdata, w270:dynamicdata, w255:dynamicdata, w273:dynamicdata, w269:dynamicdata, w256:dynamicdata, w250:dynamicdata, w268:dynamicdata)  [unwired: 15 in, 7 out]
        n130 = Or(x=w295, y=w293) -> (x .or. y?=w292:bool)
        n131 = local write "Thrust lb"(w273) -> ()
        n132 = call "Convert from Dynamic Data"("Dynamic Data Type"=w273) -> ("Array"=w297:dbl[])  [unwired: 3 in]
        n133 = call "Convert from Dynamic Data4"("Dynamic Data Type"=w268) -> ("Array"=w277:dbl[])  [unwired: 3 in]
        n134 = call "Convert from Dynamic Data3"("Dynamic Data Type"=w269) -> ("Array"=w278:dbl[])  [unwired: 3 in]
        n135 = Merge Signals(w272, w270, w255, w273, w269, w268) -> (w279:dynamicdata)
        n136 = Multiply(x=110.0, y=w250) -> (x*y=w253:dynamicdata)
        n137 = Multiply(x=200.0, y=w256) -> (x*y=w252:dynamicdata)
        n138 = Multiply(x=110.0, y=w270) -> (x*y=w271:dynamicdata)
        n139 = Subtract(1:w271, 2:w253) -> ()  [unwired: 1 in, 2 out]
        n140 = Merge Signals(w253, w252) -> (w254:dynamicdata)
        n141 = call "Convert from Dynamic Data2"("Dynamic Data Type"=w253) -> ("Array"=w258:dbl[])  [unwired: 3 in]
        n142 = call "Convert from Dynamic Data7"("Dynamic Data Type"=w252) -> ("Array"=w281:dbl[])  [unwired: 3 in]
        n143 = call-poly <vilib>:"Mean.vi"("X"=w297) -> ("mean"=w296:dbl)  [unwired: 1 out]
        n144 = call-poly <vilib>:"Mean.vi"("X"=w278) -> ("mean"=w276:dbl)  [unwired: 1 out]
        n145 = call-poly <vilib>:"Mean.vi"("X"=w277) -> ("mean"=w267:dbl)  [unwired: 1 out]
        n146 = local write "Chamber Pressure"(w271) -> ()
        n147 = call "Filter"("Signal"=w254) -> ("Filtered Signal"=w251:dynamicdata)  [unwired: 9 in, 1 out]
        n148 = Multiply(x=200.0, y=w256) -> (x*y=w259:dynamicdata)
        "Voltage Input" <- w259
        n149 = local write "Temperature"(w269) -> ()
        n150 = call-poly <vilib>:"Mean.vi"("X"=w258) -> ("mean"=w257:dbl)  [unwired: 1 out]
        "Supply Pressure Mean" <- w257
        n151 = call-poly <vilib>:"Mean.vi"("X"=w281) -> ("mean"=w280:dbl)  [unwired: 1 out]
        n152 = Multiply(x=200.0, y=w250) -> (x*y=w261:dynamicdata)
        "Test" <- w261
        n153 = call "Convert from Dynamic Data10"("Dynamic Data Type"=w259) -> ()  [unwired: 3 in, 1 out]
        n154 = Split Signals(w251) -> (w248:dynamicdata, w247:dynamicdata)  [unwired: 2 in]
        n155 = Merge Signals(w248, w247) -> (w274:dynamicdata)
        n156 = case shown="\"Cold Flow Rig\"" w298 {
          tunnel: w291 -> [w303 w307]
          tunnel: w279 -> [w300 _]
          tunnel: w274 -> [_ w306]
          frame "Test Firing", Default {
            n157 = call "Write To Measurement File3"("Signals"=w300, "Enable"="Collect Data?", "Filename"=w303) -> ("Filename Out"=→"Filename Out":path, "Saving Data"=→"Saving Data":bool, "error out"=→"error out 3":errorcluster)  [unwired: 14 in]
          }
          frame "Cold Flow Rig" {
            n158 = call "Write To Measurement File4"("Signals"=w306, "Enable"="Collect Data? 2", "Filename"=w307) -> ("Filename Out"=→"Filename Out":path, "Saving Data"=→"Saving Data":bool)  [unwired: 14 in, 1 out]
          }
        }
        n159 = call "Convert from Dynamic Data9"("Dynamic Data Type"=w261) -> ("Array"=w265:dbl[])  [unwired: 3 in]
        n160 = call-poly <vilib>:"Mean.vi"("X"=w265) -> ("mean"=w264:dbl)  [unwired: 1 out]
        n161 = local write "Supply Pressure PSI"(w248) -> ()
        n162 = local write "Mass Flow L/min"(w247) -> ()
        n163 = call "Elapsed Time"() -> ("Elapsed Time (s)"=w275:dbl)  [unwired: 12 in, 7 out]
        "Elapsed Time (s)" <- w275
        n164 = call "Convert from Dynamic Data6"("Dynamic Data Type"=w271) -> ("Array"=w283:dbl[])  [unwired: 3 in]
        n165 = call-poly <vilib>:"Mean.vi"("X"=w283) -> ("mean"=w282:dbl)  [unwired: 1 out]
        "Numeric 2" <- w299
      }
      n166 = Bundle(w27, w48) -> (→"Servo Voltage Input":cluster{dbl[], dbl[]})  [unwired: 1 in]
      n167 = Bundle(w27, w23) -> (w25:cluster{dbl[], dbl[]})  [unwired: 1 in]
      "Servo Voltage Input 2" <- w25
      n168 = Bundle(w27, w23) -> (w26:cluster{dbl[], dbl[]})  [unwired: 1 in]
      n169 = call-poly <vilib>:"Butterworth Filter.vi"("filter type"=Filter_Passband_Type."Lowpass", "low cutoff freq: fl"=25.0, "high cutoff freq: fh"=50.0, "sampling freq: fs"=60.0, "X"=w23) -> ()  [unwired: 3 in, 2 out]
      n170 = call <vilib>:"DAQmx Clear Task.vi"("task in"=w59, "error in"=w58) -> ("error out"=→"error out 2":errorcluster)  [unwired: 13 in]
      n171 = Bundle(w27, w44) -> (w41:cluster{dbl[], dbl[]})  [unwired: 1 in]
      "Supply Pressure" <- w41
      n172 = Bundle(w27, w43) -> (w40:cluster{dbl[], dbl[]})  [unwired: 1 in]
      "Chamber Pressure" <- w40
      n173 = Bundle(w27, w45) -> (w39:cluster{dbl[], dbl[]})  [unwired: 1 in]
      "MassFlow" <- w39
      n174 = Bundle(w27, w42) -> (w38:cluster{dbl[], dbl[]})  [unwired: 1 in]
      "Thrust" <- w38
      n175 = Bundle(w27, w46) -> (w37:cluster{dbl[], dbl[]})  [unwired: 1 in]
      "Temperature" <- w37
      n176 = Build Array(w25, w26) -> (→"Servo Voltage Input 3":cluster{dbl[], dbl[]}[])
      n177 = Build Array(w41, w40, w39, w38, w37) -> (→"All Channel Graph":cluster{dbl[], dbl[]}[])
    }
  }
